vi "1726 Drive With PID.vi"(0 "RobotDriveDevRef in":T1, 1 "Max Speed":dbl=0.5 min=0.0 max=1.0 step=0.05, 2 "Target Distance":dbl, 3 "Timeout (ms)":u32) -> (7 "RobotDriveDevRef out":T1, 9 "Is Finished?":bool, 10 "Is Timedout?":bool)   [LabVIEW 2016]
uses:
  <vilib>/Rock Robotics/WPI/RobotDrive/WPI_RobotDriveDevRef.ctl
  <vilib>/Rock Robotics/WPI/MotorControl/WPI_MotorControlDeviceRef.ctl
  <vilib>/Rock Robotics/WPI/MotorControl/WPI_MotorControlType.ctl
  <vilib>/Rock Robotics/SystemInterfaces/DIO/FPGA_DIOPWMChannel.ctl
  <vilib>/Rock Robotics/WPI/PWM/WPI_PWMDeadband.ctl
  <vilib>/Rock Robotics/Network Tables/NT Read Number.vi
  Team Code/Robot Global Data.vi
  <vilib>/addons/control/pid/pid.llb/PID (DBL).vi
  <vilib>/Rock Robotics/WPI/RobotDrive/WPI_RobotDriveArcadeDrive_Standard(NoSaturation).vi
  <vilib>/addons/control/pid/NI_PID_pid.lvlib
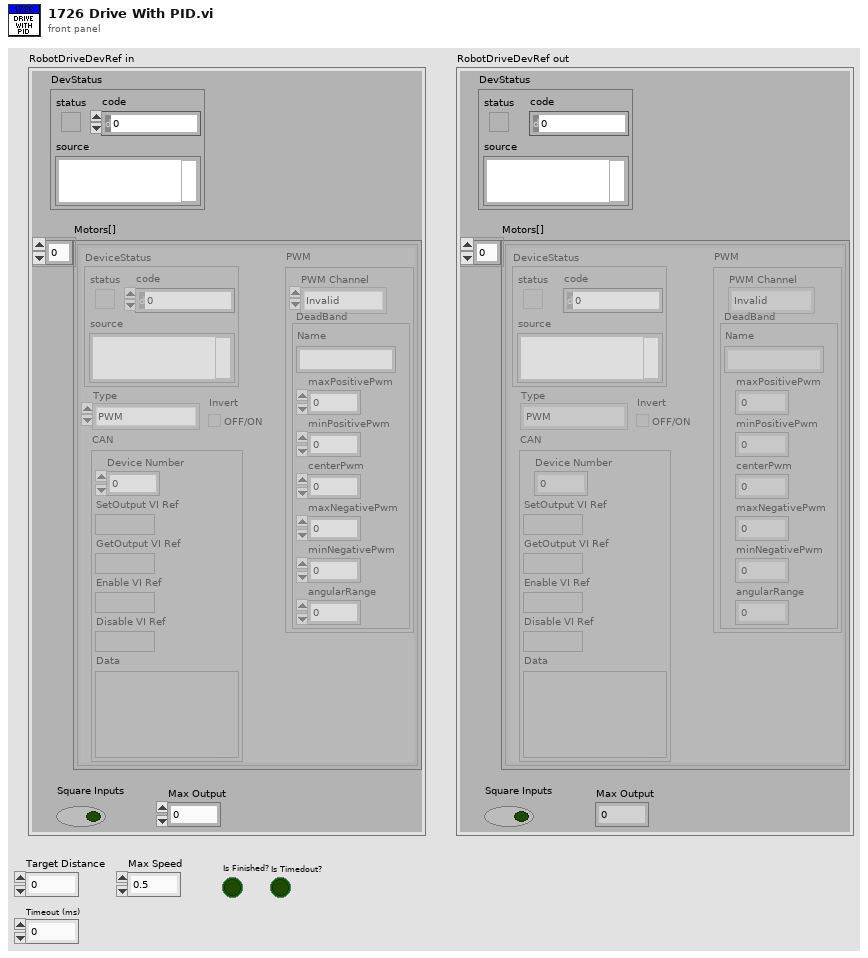
[diagram p1: front panel]
types:
  T1 = typedef "WPI_RobotDriveDevRef.ctl" = cluster{"DevStatus":errorcluster, "Motors[]":T2[], "Square Inputs":bool, "Max Output":dbl}
  T2 = typedef "WPI_MotorControlDeviceRef.ctl" = cluster{"DeviceStatus":errorcluster, "Type":T3, "PWM":cluster{"PWM Channel":T4, "DeadBand":T5}, "CAN":cluster{"Device Number":u8, "SetOutput VI Ref":variant, "GetOutput VI Ref":variant, "Enable VI Ref":variant, "Disable VI Ref":variant, "Data":variant}, "Invert":bool}
  T3 = typedef "WPI_MotorControlType.ctl" = enum16{"PWM", "CAN"}
  T4 = typedef "FPGA_DIOPWMChannel.ctl" = enum8{"PWM 0", "PWM 1", "PWM 2", "PWM 3", "PWM 4", "PWM 5", "PWM 6", "PWM 7", "PWM 8", "PWM 9", "PWM MXP 0", "PWM MXP 1", "PWM MXP 2", "PWM MXP 3", "PWM MXP 4", "PWM MXP 5", "PWM MXP 6", "PWM MXP 7", "PWM MXP 8", "PWM MXP 9", "Invalid"}
  T5 = typedef "WPI_PWMDeadband.ctl" = cluster{"Name":string, "maxPositivePwm":i32, "minPositivePwm":i32, "centerPwm":i32, "maxNegativePwm":i32, "minNegativePwm":i32, "angularRange":u16}
  T6 = cluster{"Numeric":dbl, "Numeric":dbl, "Numeric":dbl}
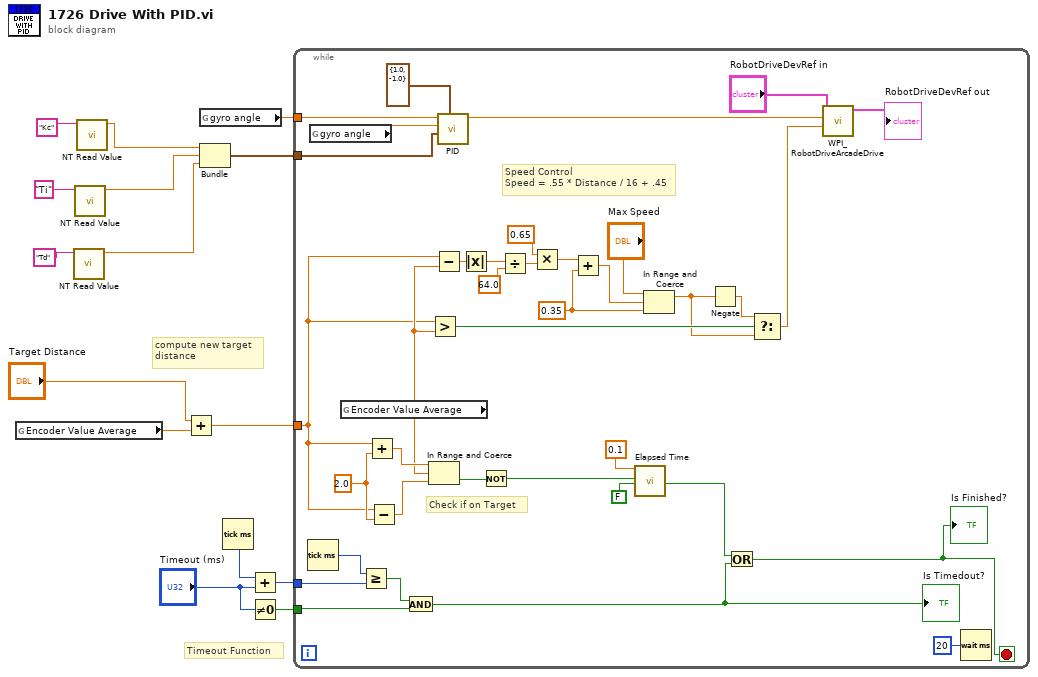
[diagram p0: block diagram]
diagram:
  # "Timeout Function"
  # "compute new target\ndistance"
  n1 = global read "Robot Global Data.vi" "Encoder Value Average"() -> (w6:dbl)
  n2 = call-poly <vilib>:"NT Read Value.vi"("Name"="Td") -> ("Numeric"=w10:dbl)  [unwired: 9 in, 1 out]
  n3 = call-poly <vilib>:"NT Read Value.vi"("Name"="Ti") -> ("Numeric"=w11:dbl)  [unwired: 9 in, 1 out]
  n4 = call-poly <vilib>:"NT Read Value.vi"("Name"="Kc") -> ("Numeric"=w12:dbl)  [unwired: 9 in, 1 out]
  n5 = Add(x="Target Distance", y=w6) -> (x+y=w5:dbl)
  n6 = global read "Robot Global Data.vi" "gyro angle"() -> (w8:dbl)
  n7 = Bundle("Numeric"=w12, "Numeric"=w11, "Numeric"=w10) -> (w9:T6)  [unwired: 1 in]
  n8 = Tick Count (ms)() -> (millisecond timer value=w4:u32)
  n9 = Add(x=w4, y="Timeout (ms)") -> (x+y=w3:u32)
  n10 = Not Equal To 0?(x="Timeout (ms)") -> (x != 0?=w1:bool)
  n11 = while {
    tunnel: w9 -> [w48]
    tunnel: w8 -> [w46]
    tunnel: w5 -> [w32]
    tunnel: w3 -> [w21]
    tunnel: w1 -> [w16]
    stop <- w19 stop-if-true
    w23 = 0.35 ("lower limit")
    w45 = 2.0 ("y")
    # "Check if on Target"
    # "Speed Control\nSpeed = .55 * Distance / 16 + .45"
    n12 = Tick Count (ms)() -> (millisecond timer value=w22:u32)
    n13 = global read "Robot Global Data.vi" "gyro angle"() -> (w47:dbl)
    n14 = global read "Robot Global Data.vi" "Encoder Value Average"() -> (w33:dbl)
    n15 = Greater Or Equal?(x=w22, y=w21) -> (x >= y?=w18:bool)
    n16 = Add(x=w32, y=w45) -> (x+y=w44:dbl)
    n17 = Subtract(x=w32, y=w45) -> (x-y=w43:dbl)
    n18 = And(x=w18, y=w16) -> (x .and. y?=w17:bool)
    "Is Timedout?" <- w17
    n19 = In Range and Coerce(upper limit=w44, x=w33, lower limit=w43) -> (In Range?=w40:bool)  [unwired: 1 out]
    n20 = Greater?(x=w32, y=w33) -> (0:w37:bool)
    n21 = Subtract(x=w32, y=w33) -> (x-y=w34:dbl)
    n22 = call-poly <vilib>:"PID.vi"("output range"=cluster{"output high":dbl, "output low":dbl} {"output high"=1.0, "output low"=-1.0}, "PID gains"=w48, "process variable"=w47, "setpoint"=w46) -> ("output"=w52:dbl)  [unwired: 6 in, 1 out]
    n23 = Absolute Value(x=w34) -> (abs(x)=w31:dbl)
    n24 = Not(x=w40) -> (.not. x?=w41:bool)
    n25 = Divide(x=w31, y=64.0) -> (x/y=w35:dbl)
    n26 = Multiply(x=0.65, y=w35) -> (x*y=w24:dbl)
    n27 = Add(x=w24, y=w23) -> (x+y=w28:dbl)
    n28 = call "Elapsed Time"("Time Target (s)"=0.1, "Reset"=w41, "Auto Reset"=FALSE) -> ("Time has Elapsed"=w20:bool)  [unwired: 9 in, 7 out]
    n29 = In Range and Coerce(upper limit="Max Speed", x=w28, lower limit=w23) -> (coerced(x)=w25:dbl)  [unwired: 1 out]
    n30 = Negate(x=w25) -> (-x=w26:dbl)
    n31 = Or(x=w20, y=w17) -> (x .or. y?=w19:bool)
    "Is Finished?" <- w19
    n32 = Select(t=w26, s=w37, f=w25) -> (s? t:f=w36:dbl)
    n33 = call-poly <vilib>:"WPI_RobotDriveArcadeDrive.vi"("Y axis value"=w36, "X axis value"=w52, "RobotDriveDevRef"="RobotDriveDevRef in") -> ("RobotDriveDevRef"=→"RobotDriveDevRef out":T1)  [unwired: 1 in, 7 out]
    n34 = Wait (ms)(milliseconds to wait=u32 20) -> ()  [unwired: 1 out]
  }
